vi "De-queue RT torque loop element.vi"(11 "RT Queues":T1) -> (0 "Data":variant, 2 "Message":string)   [LabVIEW 2018]
uses:
  Type Defs/Queues cluster.ctl
  Queues.lvlib
  Chris VIs/Message Scheduler/message scheduler.lvclass
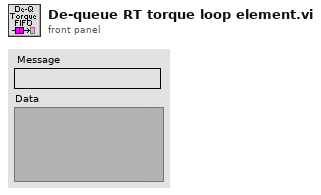
[diagram p1: front panel]
types:
  T1 = typedef "Real-Time.lvlib/Queues.lvlib/Queues cluster.ctl" = cluster{"RT Message":refnum<queue>, "RT Comms":refnum<queue>, "RT Data":refnum<queue>, "message scheduler":refnum<class "message scheduler.lvclass">}
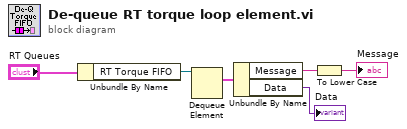
[diagram p0: block diagram]
diagram:
  n1 = Unbundle By Name("RT Queues") -> ("RT Torque FIFO"=w5:refnum<queue>)
  n2 = Dequeue Element(queue=w5) -> (element=w4:cluster{"Message":string, "Data":variant})  [unwired: 2 in, 3 out]
  n3 = Unbundle By Name(w4) -> ("Message"=w3:string, "Data"=→"Data":variant)
  n4 = To Lower Case(string=w3) -> (all lower case string=→"Message":string)
